vi "C8855_WFAVG.vi"(6 "iteration # in":i32, 8 "2D populated array in":dbl[][](array[numeric]), 9 "Input Array":u32[](array[numeric]), 10 "Number of Averages":u32, 11 "Average ON/OFF":bool) -> (0 "iteration # out":i32, 1 "2D populated array out":dbl[][](array[numeric]), 2 "Averaged Array":dbl[](array[numeric]), 3 "Average ON/OFF":bool)   [LabVIEW 2014]
uses:
  <vilib>/Analysis/baseanly.llb/Mean (DBL).vi
  <vilib>/Analysis/NI_AALBase.lvlib
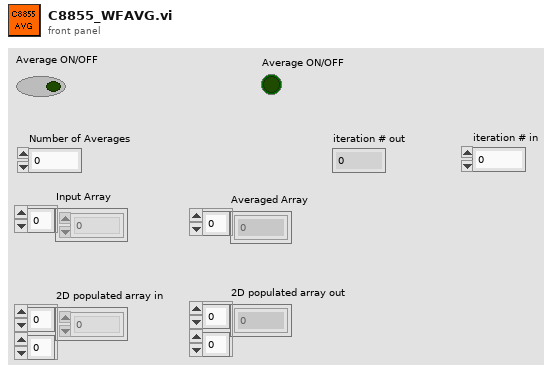
[diagram p1: front panel]
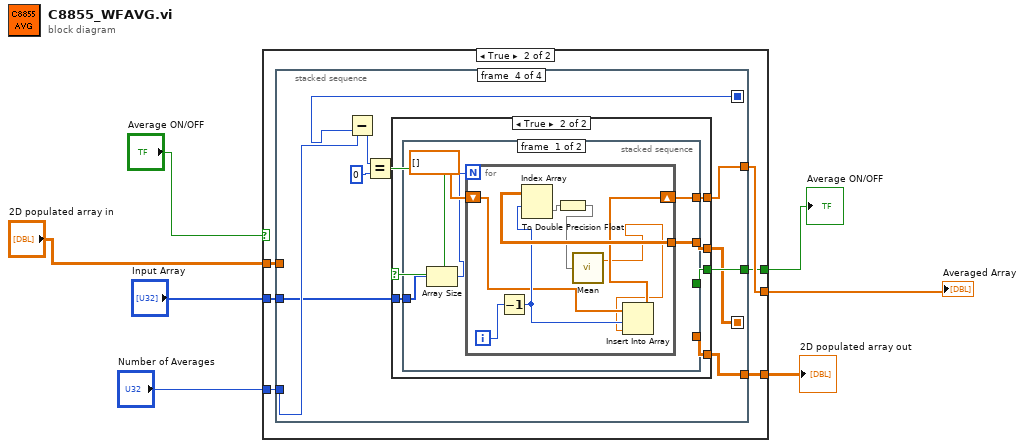
[diagram p0: block diagram]
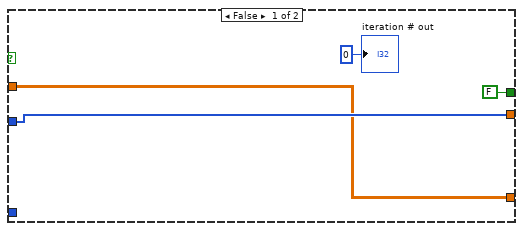
[diagram p2: hidden frame]
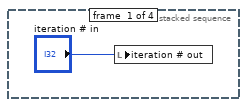
[diagram p3: hidden frame]
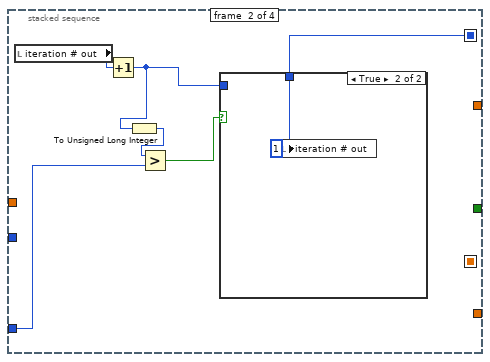
[diagram p4: hidden frame]
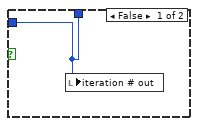
[diagram p5: hidden frame]
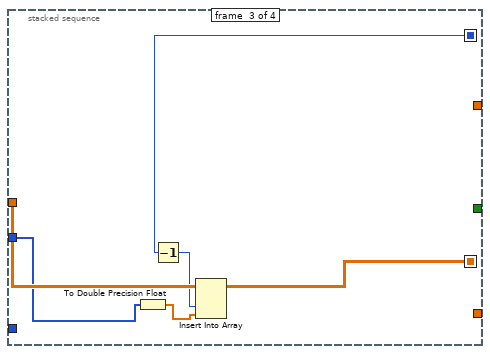
[diagram p6: hidden frame]
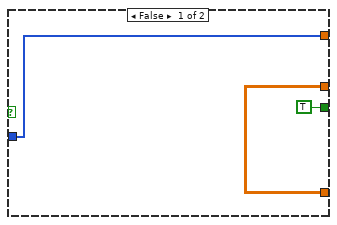
[diagram p7: hidden frame]
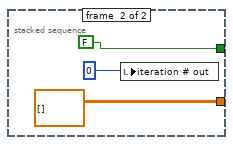
[diagram p8: hidden frame]
diagram:
  n1 = case shown="True" "Average ON/OFF" {
    tunnel: "Input Array" -> [w10 w17]
    tunnel: "2D populated array in" -> [w9 w16]
    tunnel: [w10 w15] -> w1
    tunnel: [w9 w12] -> w4
    tunnel: "Number of Averages" -> [_ w14]
    tunnel: [FALSE ("Average ON/OFF") w13] -> w2
    frame False {
      "iteration # out" <- 0 ("iterations")
    }
    frame True {
      n2 = stacked-sequence {
        seq-local: [_ _ w31 _] -> [_ _ _ w41]
        seq-local: [_ w19 _ _] -> [_ _ w30 w36]
        tunnel: w17 -> [_ _ w29 w34]
        tunnel: w16 -> [_ _ w32 _]
        tunnel: [_ _ _ w33] -> w15
        tunnel: w14 -> [_ w24 _ w39]
        tunnel: [_ _ _ w42] -> w13
        tunnel: [_ _ _ w40] -> w12
        frame #0 {
          n3 = local write "iteration # out"("iteration # in") -> ()
        }
        frame #1 {
          n4 = local read "iteration # out"() -> (w21:i32)
          n5 = Increment(x=w21) -> (x+1=w20:i32)
          n6 = To Unsigned Long Integer(number=w20) -> (unsigned 32bit integer=w23:u32)
          n7 = Greater?(x=w23, y=w24) -> (0:w22:bool)
          n8 = case shown="True" w22 {
            tunnel: w20 -> [w25 _]
            tunnel: [w25 w26] -> w19
            frame False {
              n9 = local write "iteration # out"(w25) -> ()
            }
            frame True {
              w26 = 1 ("iterations")
              n10 = local write "iteration # out"(w26) -> ()
            }
          }
        }
        frame #2 {
          n11 = To Double Precision Float(number=w29) -> (double precision float=w28:dbl[])
          n12 = Decrement(x=w30) -> (x-1=w27:i32)
          n13 = Insert Into Array(array=w32, index (col)=w27, new element=w28) -> (w31:dbl[][])  [unwired: 1 in]
        }
        frame #3 {
          n14 = Subtract(x=w39, y=w36) -> (x-y=w35:u32)
          n15 = Equal?(x=w35, y=0) -> (x = y?=w37:bool)
          n16 = case shown="True" w37 {
            tunnel: [TRUE ("Average ON/OFF") w50] -> w42
            tunnel: [w44 w49] -> w40
            tunnel: w41 -> [w44 w48]
            tunnel: w34 -> [w43 w47]
            tunnel: [w43 w46] -> w33
            frame False {
            }
            frame True {
              n17 = stacked-sequence {
                tunnel: [_ FALSE ("Average ON/OFF")] -> w50
                tunnel: [_ dbl[][] [] ("2D populated array in")] -> w49
                tunnel: w48 -> [w55 _]
                tunnel: w47 -> [w53 _]
                tunnel: [w51 _] -> w46
                frame #0 {
                  n18 = Array Size(array=w53) -> (size(s)=w52:i32)
                  n19 = for {
                    N: w52 -> [_]
                    tunnel: w55 -> [w62]
                    shift-right: [w58] -> w51
                    shift-left: dbl[] [] -> [w57]
                    i -> [w63]
                    n20 = Decrement(x=w63) -> (x-1=w61:i32)
                    n21 = Index Array(array=w62, index (row)=w61) -> (element=w60:dbl[])  [unwired: 1 in]
                    n22 = To Double Precision Float(number=w60) -> (double precision float=w59:dbl[])
                    n23 = call-poly <vilib>:"Mean.vi"("X"=w59) -> ("mean"=w56:dbl)  [unwired: 1 out]
                    n24 = Insert Into Array(array=w57, index=w61, new element=w56) -> (w58:dbl[])
                  }
                }
                frame #1 {
                  n25 = local write "iteration # out"(0 ("iterations")) -> ()
                }
              }
            }
          }
        }
      }
    }
  }
  "Averaged Array" <- w1
  "2D populated array out" <- w4
  "Average ON/OFF" <- w2
